vi "Next Step.vi"(8 "error in (no error)":errorcluster, 11 "Magna Voltage Scan in":refnum<class "Magna Voltage Scan.lvclass">) -> (0 "error out":errorcluster, 1 "Current Step":u32, 2 "Current Position":dbl, 3 "Magna Voltage Scan out":refnum<class "Magna Voltage Scan.lvclass">)   [LabVIEW 2012, in "Magna Voltage Scan.lvclass"]
doc: "(Dynamic) Move to the next preconfigured step of this Scanner, and return the current position (actual, not intended) of this Scanner. Increment the step counter by one."
uses:
  Magna Voltage Scan.lvclass
  Instruments/Magna-Power Power Supply/Magna Power.lvclass
  Scanner/Scanner.lvclass
  Magna Voltage Scan.lvclass/Magna Voltage Scan.ctl
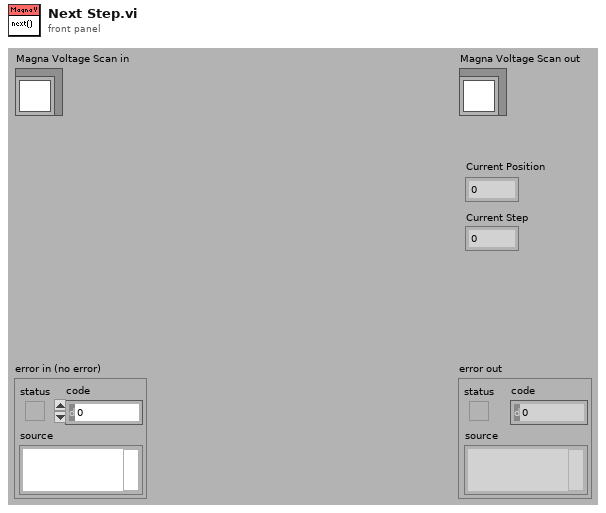
[diagram p1: front panel]
types:
  T1 = typedef "Scanner.lvclass/Range.ctl" = cluster{"xi":dbl, "xf":dbl, "dx":dbl, "Return to...?":bool, "Return to":dbl}
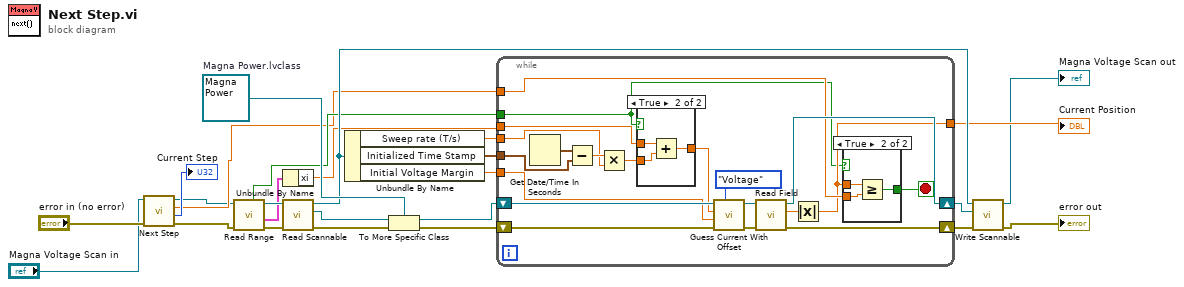
[diagram p0: block diagram]
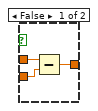
[diagram p2: hidden frame]
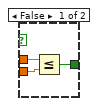
[diagram p3: hidden frame]
diagram:
  w20 = refnum<class "Magna Power.lvclass"> refnum  # Magna Power.lvclass
  n1 = call-parent "Next Step.vi"("error in (no error)"="error in (no error)", "Scanner in"="Magna Voltage Scan in") -> ("error out"=w4:errorcluster, "Current Step"=→"Current Step":u32, "Current Position"=w6:dbl, "Scanner out"=w5:refnum<class "Magna Voltage Scan.lvclass">)  [unwired: 6 in]
  n2 = call-dynamic "Read Range.vi"("error in (no error)"=w4, "Scanner.lvclass in"=w5) -> ("error out"=w19:errorcluster, "Range"=w17:T1, "Scanner.lvclass out"=w18:refnum<class "Magna Voltage Scan.lvclass">, "Scanning Up?"=w9:bool)  [unwired: 4 in, 2 out]
  n3 = Unbundle By Name(w17) -> ("xi"=w8:dbl)
  n4 = call-dynamic "Read Scannable.vi"("error in (no error)"=w19, "Scanner.lvclass in"=w18) -> ("error out"=w22:errorcluster, "Scannable.lvclass"=w21:refnum<class "Scannable.lvclass">, "Scanner.lvclass out"=w10:refnum<class "Magna Voltage Scan.lvclass">)  [unwired: 7 in]
  n5 = Unbundle By Name(w10) -> ("Sweep rate (T/s)"=w15:dbl, "Initialized Time Stamp"=w16:timestamp, "Initial Voltage Margin"=w7:dbl)
  n6 = To More Specific Class(target class=w20, reference=w21, error in=w22) -> (specific class reference=w13:refnum<class "Magna Power.lvclass">, error out=w14:errorcluster)
  n7 = while {
    tunnel: w16 -> [w44]
    tunnel: w15 -> [w42]
    shift-right: [w35] -> w12
    shift-left: w14 -> [w41]
    shift-right: [w36] -> w11
    shift-left: w13 -> [w40]
    tunnel: w9 -> [w30]
    tunnel: w6 -> [w34]
    tunnel: [w31] -> w3
    tunnel: w8 -> [w29]
    tunnel: w7 -> [w27]
    stop <- w33 stop-if-true
    n8 = Get Date/Time In Seconds() -> (seconds since 1Jan1904=w45:timestamp)
    n9 = Subtract(x=w45, y=w44) -> (x-y=w43:dbl)
    n10 = Multiply(x=w43, y=w42) -> (x*y=w28:dbl)
    n11 = case shown="True" w30 {
      tunnel: [w48 w51] -> w39
      tunnel: w29 -> [w47 w50]
      tunnel: w28 -> [w46 w49]
      frame False {
        n12 = Subtract(x=w47, y=w46) -> (x-y=w48:dbl)
      }
      frame True {
        n13 = Add(x=w50, y=w49) -> (x+y=w51:dbl)
      }
    }
    n14 = call "Guess Current With Offset.vi"("V or I?"=enum16{"Voltage", "Current"}."Voltage", "error in (no error)"=w41, "Offset"=w27, "Desired Field"=w39, "Magna Power in"=w40) -> ("error out"=w38:errorcluster, "Magna Power out"=w37:refnum<class "Magna Power.lvclass">)  [unwired: 4 in, 1 out]
    n15 = call "Read Field.vi"("error in (no error)"=w38, "Magna Power in"=w37) -> ("error out"=w35:errorcluster, "Field (T)"=w32:dbl, "Magna Power out"=w36:refnum<class "Magna Power.lvclass">)  [unwired: 5 in, 2 out]
    n16 = Absolute Value(x=w32) -> (abs(x)=w31:dbl)
    n17 = case shown="True" w30 {
      tunnel: w31 -> [w54 w55]
      tunnel: w34 -> [w53 w57]
      tunnel: [w52 w56] -> w33
      frame False {
        n18 = Less Or Equal?(x=w54, y=w53) -> (x <= y?=w52:bool)
      }
      frame True {
        n19 = Greater Or Equal?(x=w55, y=w57) -> (x >= y?=w56:bool)
      }
    }
  }
  "Current Position" <- w3
  n20 = call-dynamic "Write Scannable.vi"("error in (no error)"=w12, "Scannable.lvclass"=w11, "Scanner.lvclass in"=w10) -> ("error out"=→"error out":errorcluster, "Scanner.lvclass out"=→"Magna Voltage Scan out":refnum<class "Magna Voltage Scan.lvclass">)  [unwired: 7 in]
